vi "Counter_Clear.vi"() -> (0 "output cluster":T1)   [LabVIEW 2010]
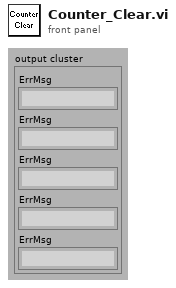
[diagram p1: front panel]
types:
  T1 = cluster{"ErrMsg":string, "ErrMsg":string, "ErrMsg":string, "ErrMsg":string, "ErrMsg":string}
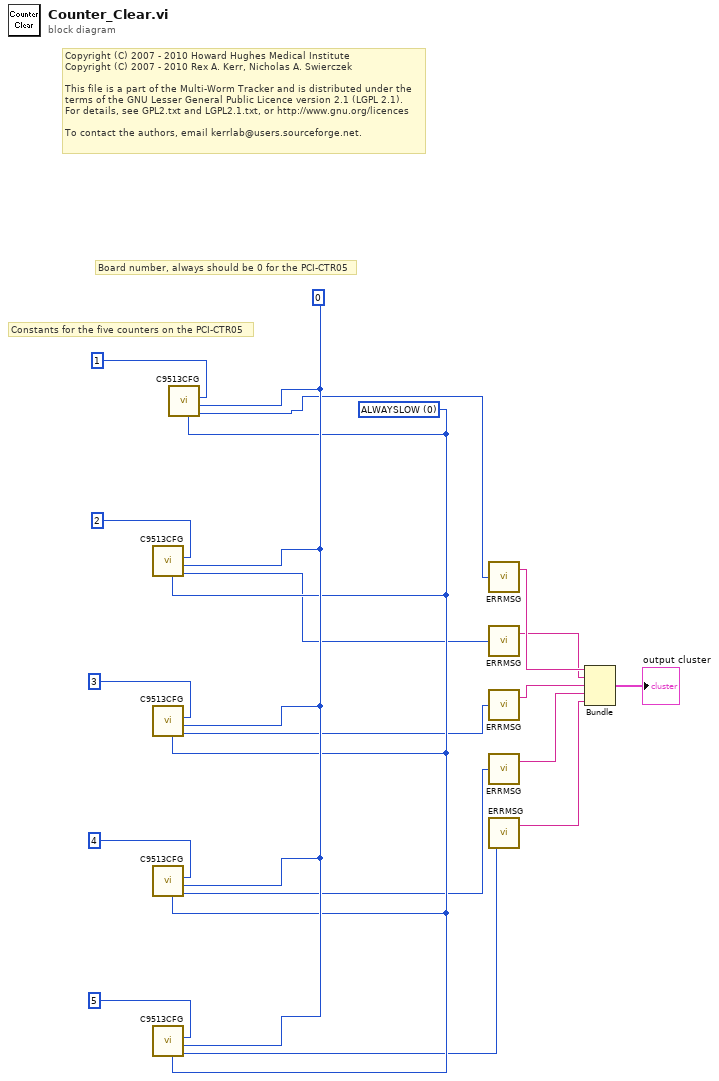
[diagram p0: block diagram]
diagram:
  w17 = u32 0 items=["ALWAYSLOW", "HIGHPULSEONTC", "TOGGLEONTC", "DISCONNECTED", "LOWPULSEONTC"] ("OutputControl (LOW)")
  w18 = u32 0 ("BoardNum (0)")
  # "Copyright (C) 2007 - 2010 Howard Hughes Medical Institute\nCopyright (C) 2007 - 2010 Rex A. Kerr, Nicholas A. Swierczek\n \nThis file is a part of the Multi-Worm Tracker and is distributed under the\nterms of the GNU Lesser General Public Licence version 2.1 (LGPL 2.1).\nFor details, see GPL2.txt and LGPL2.1.txt, or http://www.gnu.org/licences\n \nTo contact the authors, email kerrlab@users.sourceforge.net."
  # "Constants for the five counters on the PCI-CTR05"
  # "Board number, always should be 0 for the PCI-CTR05"
  n1 = call <menus>:"C9513CFG.VI"("OutputControl (LOW)"=w17, "BoardNum (0)"=w18, "CounterNum (1)"=u32 2) -> ("ErrCode"=w9:i32)  [unwired: 8 in]
  n2 = call <menus>:"C9513CFG.VI"("OutputControl (LOW)"=w17, "BoardNum (0)"=w18, "CounterNum (1)"=u32 3) -> ("ErrCode"=w8:i32)  [unwired: 8 in]
  n3 = call <menus>:"C9513CFG.VI"("OutputControl (LOW)"=w17, "BoardNum (0)"=w18, "CounterNum (1)"=u32 4) -> ("ErrCode"=w7:i32)  [unwired: 8 in]
  n4 = call <menus>:"C9513CFG.VI"("OutputControl (LOW)"=w17, "BoardNum (0)"=w18, "CounterNum (1)"=u32 5) -> ("ErrCode"=w6:i32)  [unwired: 8 in]
  n5 = call <menus>:"C9513CFG.VI"("OutputControl (LOW)"=w17, "BoardNum (0)"=w18, "CounterNum (1)"=u32 1) -> ("ErrCode"=w10:i32)  [unwired: 8 in]
  n6 = call <menus>:"ERRMSG.VI"("ErrCode"=w10) -> ("ErrMsg"=w16:string)  [unwired: 1 out]
  n7 = call <menus>:"ERRMSG.VI"("ErrCode"=w9) -> ("ErrMsg"=w15:string)  [unwired: 1 out]
  n8 = call <menus>:"ERRMSG.VI"("ErrCode"=w8) -> ("ErrMsg"=w14:string)  [unwired: 1 out]
  n9 = call <menus>:"ERRMSG.VI"("ErrCode"=w7) -> ("ErrMsg"=w13:string)  [unwired: 1 out]
  n10 = call <menus>:"ERRMSG.VI"("ErrCode"=w6) -> ("ErrMsg"=w12:string)  [unwired: 1 out]
  n11 = Bundle("ErrMsg"=w16, "ErrMsg"=w15, "ErrMsg"=w14, "ErrMsg"=w13, "ErrMsg"=w12) -> (→"output cluster":T1)  [unwired: 1 in]
